vi "LOGIC_set_imname.vi"(11 "Database RefNum in":T1) -> (2 "imname":string)   [LabVIEW 2016]
uses:
  DBSHAND/private/vis/DatabaseHand_RefNum.ctl
  DBSHAND/private/vis/DatabaseHand_Element_Get(string).vi
  DBSHAND/private/vis/DatabaseHand_Element_Get(I32).vi
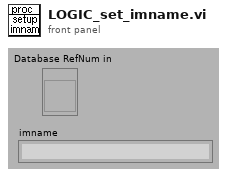
[diagram p1: front panel]
types:
  T1 = typedef "DatabaseHand_RefNum.ctl" = refnum<vi>
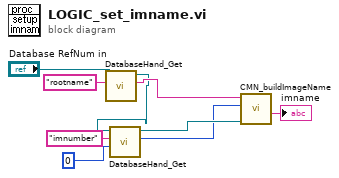
[diagram p0: block diagram]
diagram:
  n1 = call-poly "DatabaseHand_Get.vi"("name"="rootname", "Database RefNum in"="Database RefNum in") -> ("value"=w7:string, "Database RefNum out"=w6:T1)  [unwired: 3 in, 5 out]
  n2 = call-poly "DatabaseHand_Get.vi"("default value"=0, "name"="imnumber", "Database RefNum in"=w6) -> ("value"=w3:i32, "Database RefNum out"=w8:T1)  [unwired: 2 in, 5 out]
  n3 = call "CMN_buildImageName.vi"("Database RefNum out"=w8, "imageNumber"=w3, "root name"=w7) -> ("image"=→"imname":string)  [unwired: 1 in, 5 out]
